vi "Derivering.vi"(1 "Input Array Y":dbl[](array[numeric]), 2 "Input Array X":dbl[](array[numeric])) -> (0 "Output Array":dbl[](array[numeric]))   [LabVIEW 2016]
panel:
  out "x-y":dbl
  out "x-y 2":dbl
  out "Waveform Graph":dbl[](graph)
  out "Waveform Graph 2":dbl[](graph)
  out "Waveform Graph 3":dbl[](graph)
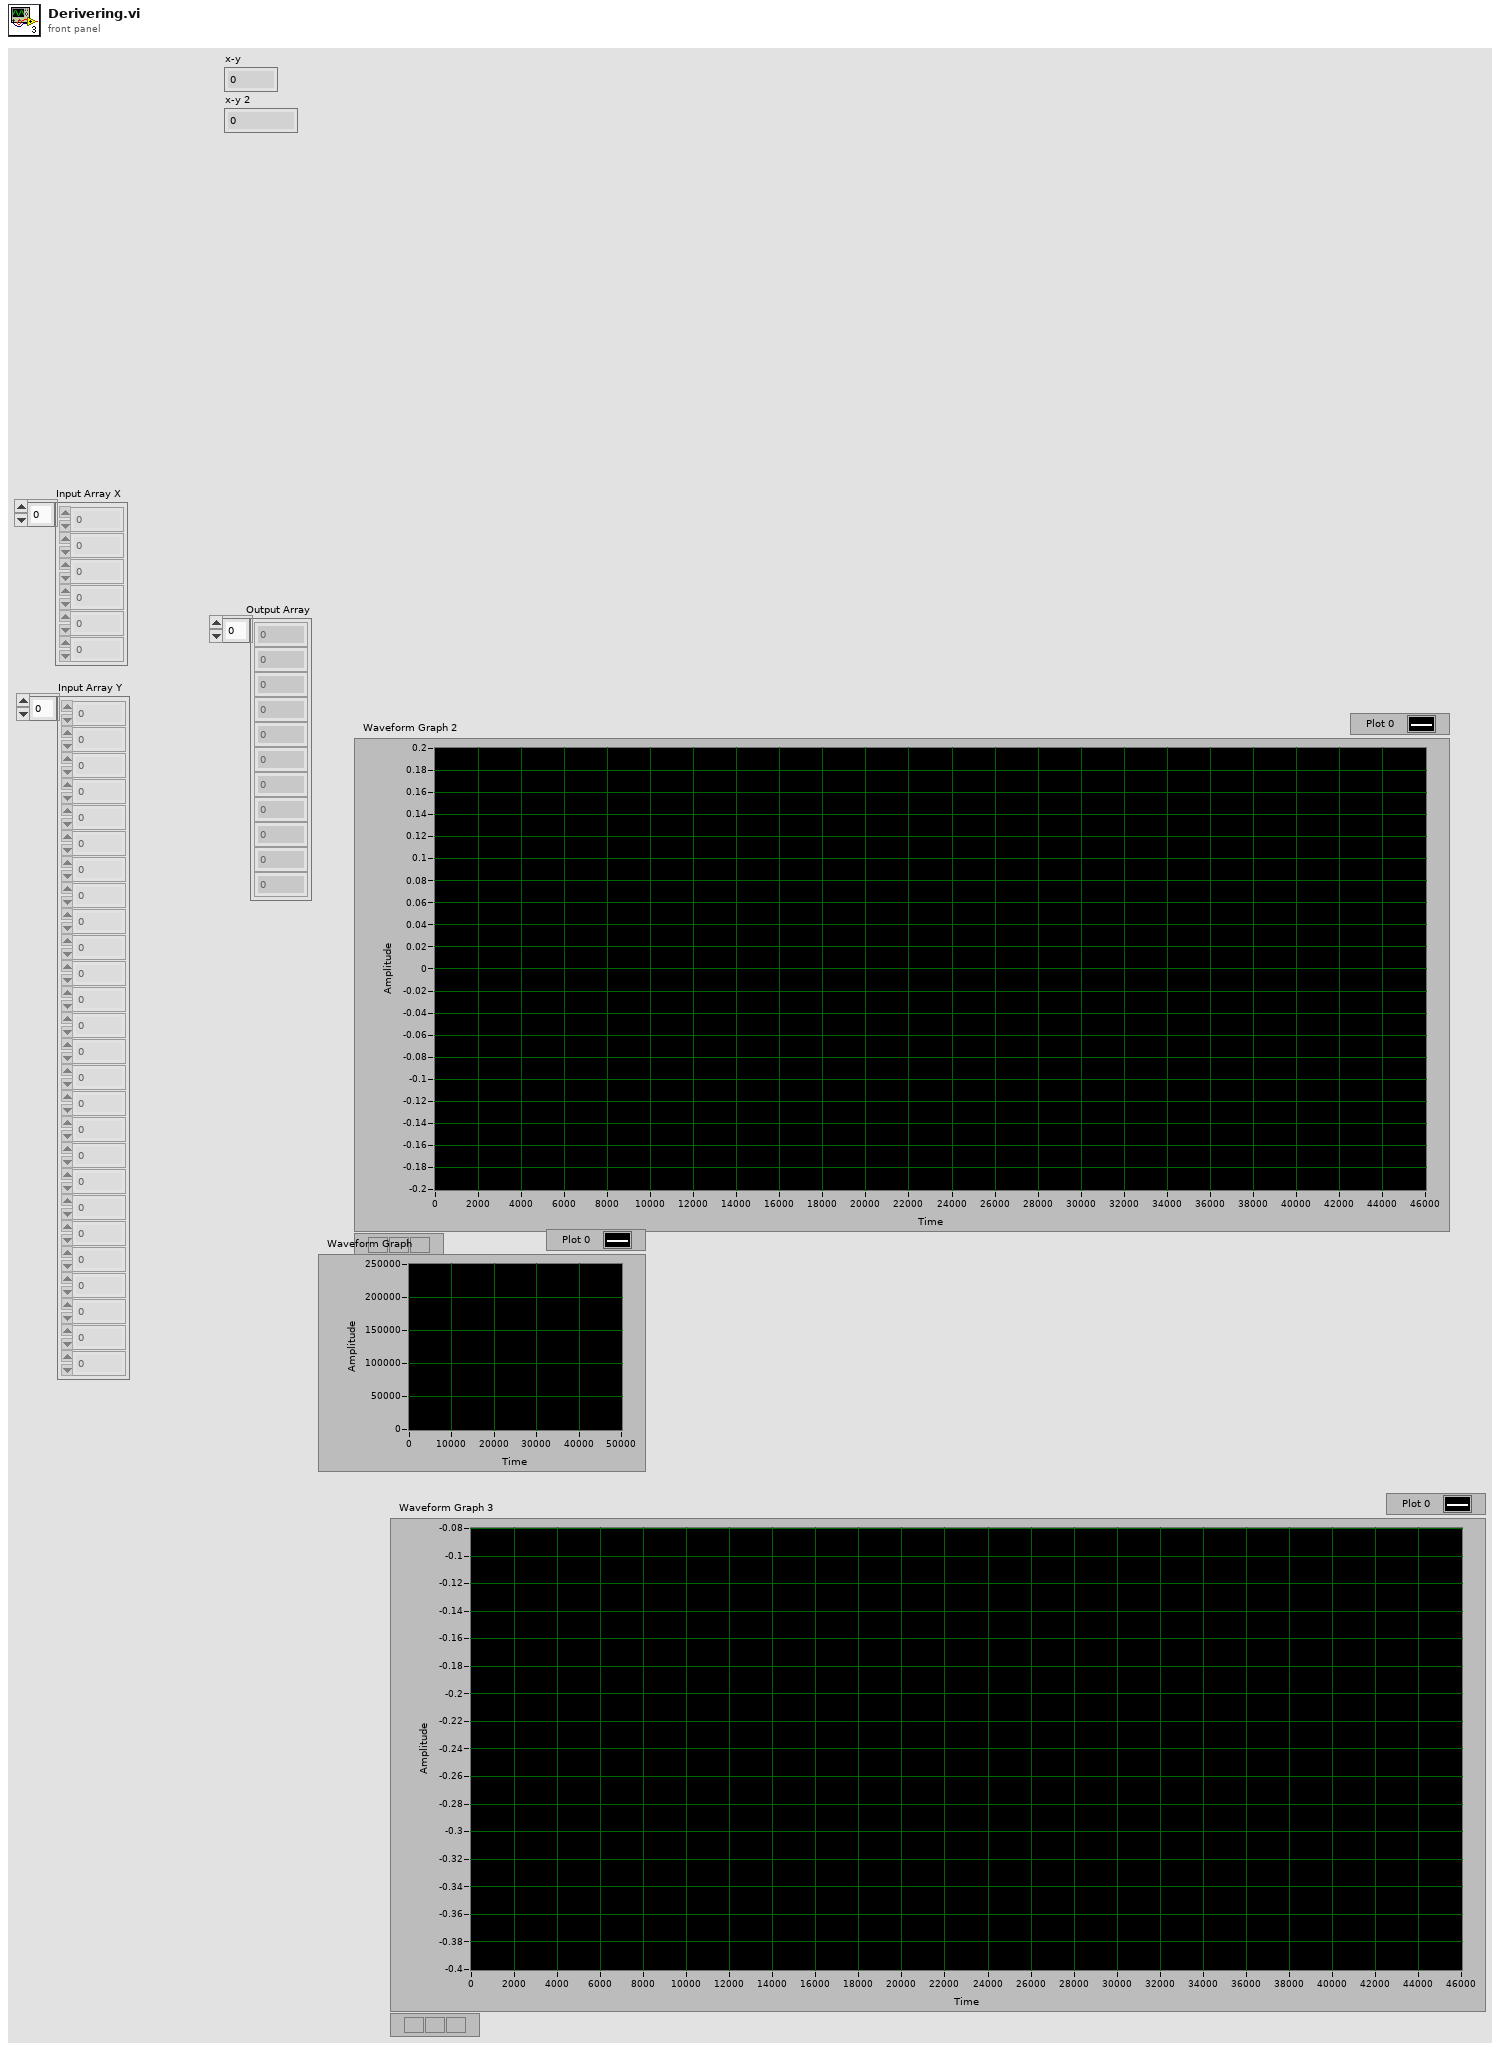
[diagram p1: front panel]
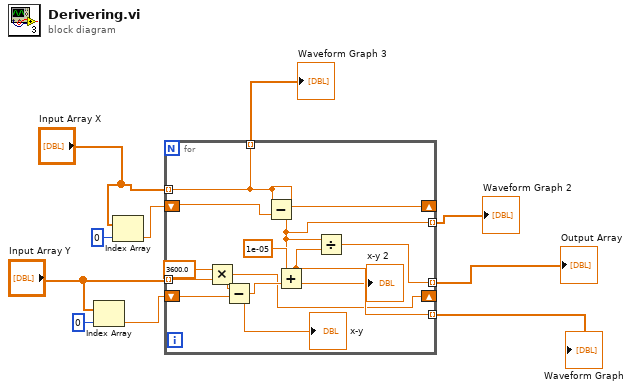
[diagram p0: block diagram]
diagram:
  n1 = Index Array(array="Input Array Y", index=0) -> (element=w7:dbl)
  n2 = Index Array(array="Input Array X", index=0) -> (element=w6:dbl)
  n3 = for {
    shift-right: [w12] -> _
    shift-left: w7 -> [w21]
    tunnel: "Input Array Y" -> [w17] mode=indexing
    tunnel: "Input Array X" -> [w13] mode=indexing
    shift-right: [w13] -> _
    shift-left: w6 -> [w20]
    tunnel: [w18] -> w1 mode=indexing
    tunnel: [w15] -> w8 mode=indexing
    tunnel: [w14] -> w9 mode=indexing
    tunnel: [w13] -> w10 mode=indexing
    n4 = Multiply(x=3600.0, y=w17) -> (x*y=w12:dbl)
    n5 = Subtract(x=w12, y=w21) -> (x-y=w19:dbl)
    "x-y" <- w19
    n6 = Subtract(x=w13, y=w20) -> (x-y=w14:dbl)
    "x-y 2" <- w14
    n7 = Add(x=1e-05, y=w19) -> (x+y=w15:dbl)
    n8 = Divide(x=w14, y=w15) -> (x/y=w18:dbl)
  }
  "Output Array" <- w1
  "Waveform Graph" <- w8
  "Waveform Graph 2" <- w9
  "Waveform Graph 3" <- w10
